vi "3ph Power from 9239 (DAQmx).vi"(5 "PTO1 Summary":refnum<queue>, 7 "PTO1 TDMS":refnum<queue>, 8 "error in":errorcluster, 10 "3ph Inputs":T1={"voltage channels"="Mod3/ai0:2", "minimum voltage value"=-10.0, "maximum voltage value"=10.0, "3ph sample rate [Hz]"=5000.0, "3phf samples per channel"=500, "Voltage Scaling"=100.0, "Current Scaling"=100.0} {"Current Scaling" format="%0.2f"; "Voltage Scaling" format="%0.2f"; "3phf samples per channel" format="%0.2f"; "3ph sample rate [Hz]" format="%0.2f"; "maximum voltage value" format="%0.2f"; "minimum voltage value" format="%0.2f"}, 11 "Queue in":refnum<queue>) -> (0 "error out":errorcluster)   [LabVIEW 2019]
doc: "Demonstrates how to implement basic power measurement on a three-phase electrical power system, such as power and energy values, frequency amplitudes, and symmetrical components."
uses:
  3ph Inputs.ctl
  Globals and Definitions/System Message.ctl
  <vilib>/DAQmx/read.llb/DAQmx Read (Analog 1D Wfm NChan NSamp).vi
  <vilib>/DAQmx/create/channels.llb/DAQmx Create Channel (AI-Voltage-Basic).vi
  <vilib>/DAQmx/configure/timing.llb/DAQmx Timing (Sample Clock).vi
  Globals and Definitions/Initialization Globals.vi
  Globals and Definitions/RT Globals RD v1.0.vi
  <vilib>/DAQmx/miscellaneous.llb/DAQmx Fill In Error Info.vi
  Globals and Definitions/Control Globals RD v1.0.vi
  <vilib>/addons/Electrical Power/Basic/Measurement/Frequency (N Channels).vi
  <vilib>/addons/Electrical Power/Basic/Measurement/RMS (N Channels).vi
  <vilib>/addons/Electrical Power/Basic/Measurement/Power (N Channels).vi
  <vilib>/addons/Electrical Power/Basic/Measurement/Energy (N Channels).vi
  <vilib>/addons/Electrical Power/Basic/NI_EP_Basic.lvlib
  <resource>/objmgr/daqmx.rc
panel:
  out "Current":waveform(dbl)[](graph)
  out "Voltages":waveform(dbl)[](graph)
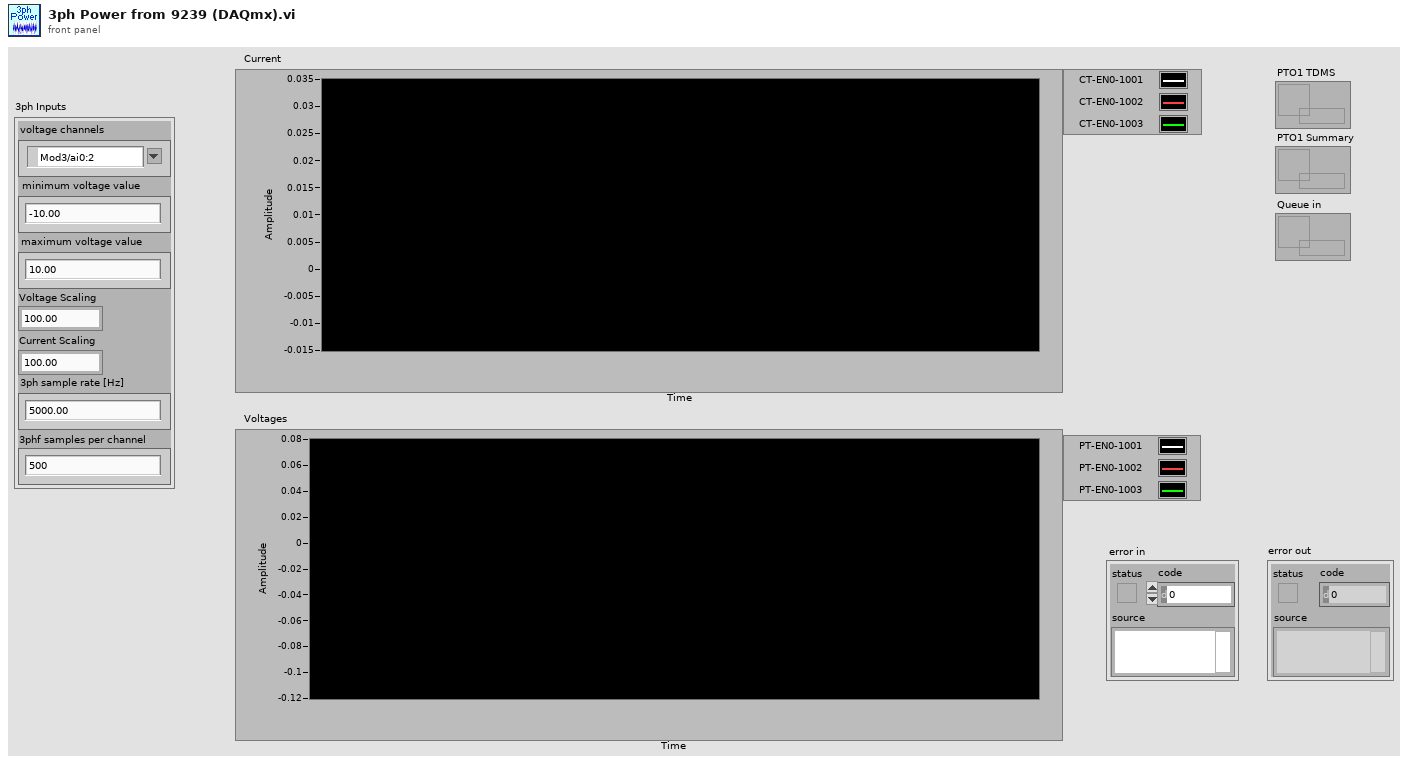
[diagram p1: front panel]
types:
  T1 = typedef "3ph Inputs.ctl" = cluster{"voltage channels":tag, "minimum voltage value":dbl, "maximum voltage value":dbl, "3ph sample rate [Hz]":dbl, "3phf samples per channel":i32, "Voltage Scaling":dbl, "Current Scaling":dbl}
  T2 = typedef "NI_EP_Basic.lvlib/basic_Power Value.ctl" = cluster{"active power [W]":dbl, "apparent power [VA]":dbl, "reactive power [VAR]":dbl, "power factor":dbl}
  T3 = typedef "NI_EP_Basic.lvlib/basic_Energy Value.ctl" = cluster{"active energy [Wh]":dbl, "apparent energy [VAh]":dbl, "reactive energy [VARh]":dbl}
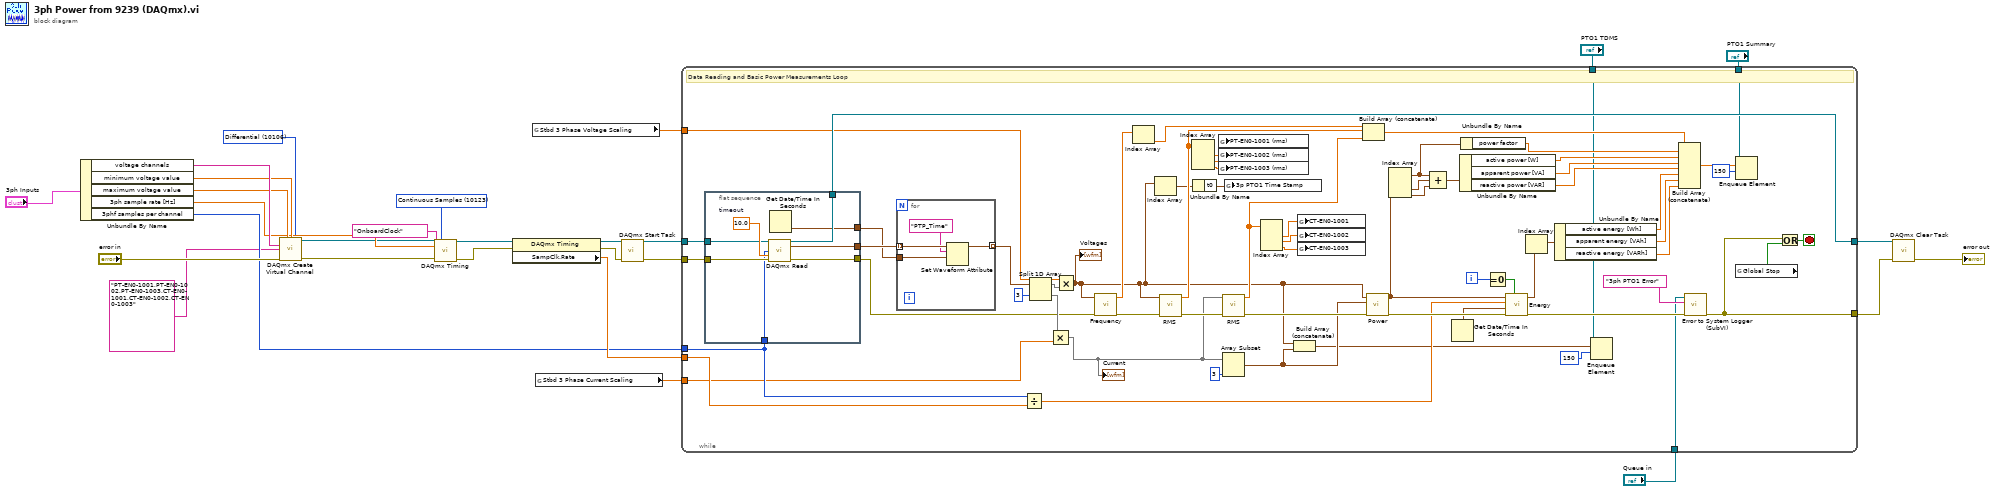
[diagram p0: block diagram]
diagram:
  w10 = 10106 items=["Default"=-1, "RSE"=10083, "NRSE"=10078, "Differential"=10106, "Pseudodifferential"=12529] ("input terminal configuration")
  w26 = 10123 items=["Finite Samples"=10178, "Continuous Samples"=10123] ("sample mode")
  n1 = Unbundle By Name("3ph Inputs") -> ("voltage channels"=w17:tag, "minimum voltage value"=w16:dbl, "maximum voltage value"=w15:dbl, "3ph sample rate [Hz]"=w14:dbl, "3phf samples per channel"=w13:i32)
  n2 = call-poly <vilib>:"DAQmx Create Virtual Channel.vi"("maximum value"=w15, "minimum value"=w16, "input terminal configuration"=w10, "physical channels"=w17, "name to assign"="PT-EN0-1001,PT-EN0-1002,PT-EN0-1003,CT-EN0-1001,CT-EN0-1002,CT-EN0-1003", "error in"="error in") -> ("task out"=w12:refnum<k21>, "error out"=w11:errorcluster)  [unwired: 8 in]
  n3 = call-poly <vilib>:"DAQmx Timing.vi"("task/channels in"=w12, "sample mode"=w26, "rate"=w14, "source"=tag "OnboardClock", "error in"=w11) -> ("task out"=w24:refnum<k21>, "error out"=w22:errorcluster)  [unwired: 9 in]
  n4 = property class="DAQmx Timing"(reference=w24, error in=w22) -> (reference out=w23:refnum<k21>, error out=w21:errorcluster, "SampClk.Rate"=w20:dbl)
  n5 = global read "Initialization Globals.vi" "Stbd 3 Phase Voltage Scaling"() -> (w8:dbl[])
  n6 = global read "Initialization Globals.vi" "Stbd 3 Phase Current Scaling"() -> (w7:dbl[])
  n7 = call <vilib>:"DAQmx Start Task.vi"("task/channels in"=w23, "error in"=w21) -> ("task out"=w28:refnum<k21>, "error out"=w25:errorcluster)  [unwired: 12 in]
  n8 = while {
    tunnel: w28 -> [w38]
    tunnel: [w91] -> w27
    tunnel: w20 -> [w60]
    tunnel: w13 -> [w59]
    tunnel: w8 -> [w32]
    tunnel: w7 -> [w48]
    tunnel: "PTO1 Summary" -> [w46]
    tunnel: "PTO1 TDMS" -> [w39]
    tunnel: w25 -> [w92]
    tunnel: "Queue in" -> [w40]
    tunnel: [w29] -> w1
    i -> [w58]
    stop <- w93 stop-if-true
    # "Data Reading and Basic Power Measurements Loop"
    n9 = flat-sequence {
      tunnel: w92 -> [w101]
      tunnel: [w100] -> w91
      tunnel: [w95] -> w35
      tunnel: [w98] -> w61
      tunnel: w59 -> [w97]
      tunnel: w38 -> [w96]
      tunnel: [w94] -> w31
      frame #0 {
        w99 = 10.0  # timeout
        n10 = call-poly <vilib>:"DAQmx Read.vi"("task/channels in"=w96, "number of samples per channel"=w97, "timeout"=w99, "error in"=w101) -> ("task out"=w100:refnum<k21>, "data"=w95:waveform(dbl)[], "error out"=w98:errorcluster)  [unwired: 9 in]
        n11 = Get Date/Time In Seconds() -> (seconds since 1Jan1904=w94:timestamp)
      }
    }
    n12 = for {
      tunnel: w35 -> [w105] mode=indexing
      tunnel: w31 -> [w104]
      tunnel: [w103] -> w30 mode=indexing
      n13 = Set Waveform Attribute(5:w104, 6:"PTP_Time" ("name"), 7:w105) -> (3:w103:waveform(dbl))  [unwired: 1 in, 2 out]
    }
    n14 = Divide(x=w59, y=w60) -> (x/y=w85:dbl)
    n15 = Split 1D Array(array=w30, index=3) -> (first subarray=w80:waveform(dbl)[], second subarray=w79:waveform(dbl)[])
    n16 = Multiply(x=w79, y=w48) -> (x*y=w33:waveform(dbl)[])
    "Current" <- w33
    n17 = Multiply(x=w32, y=w80) -> (x*y=w34:waveform(dbl)[])
    "Voltages" <- w34
    n18 = call-poly <vilib>:"Frequency.vi"("error in (no error)"=w61, "waveforms"=w34) -> ("error out"=w90:errorcluster, "frequencies"=w89:dbl[])  [unwired: 8 in]
    n19 = Index Array(array=w89) -> (element=w74:dbl)  [unwired: 1 in]
    n20 = Index Array(array=w34) -> (element=w53:waveform(dbl))  [unwired: 1 in]
    n21 = call-poly <vilib>:"RMS.vi"("error in (no error)"=w90, "waveforms"=w34) -> ("error out"=w83:errorcluster, "RMS values"=w54:dbl[])  [unwired: 8 in]
    n22 = Index Array(array=w54) -> (element #1=w57:dbl, element #2=w56:dbl, element #3=w55:dbl)  [unwired: 3 in]
    n23 = Unbundle By Name(w53) -> ("t0"=w47:timestamp)
    n24 = global write "Control Globals RD v1.0.vi" "PT-EN0-1001 (rms)"(w57) -> ()
    n25 = global write "Control Globals RD v1.0.vi" "PT-EN0-1002 (rms)"(w56) -> ()
    n26 = global write "Control Globals RD v1.0.vi" "PT-EN0-1003 (rms)"(w55) -> ()
    n27 = Array Subset(array=w33, length=3) -> (w78:waveform(dbl)[])  [unwired: 1 in]
    n28 = call-poly <vilib>:"RMS.vi"("error in (no error)"=w83, "waveforms"=w33) -> ("error out"=w82:errorcluster, "RMS values"=w49:dbl[])  [unwired: 8 in]
    n29 = global write "Control Globals RD v1.0.vi" "3p PTO1 Time Stamp"(w47) -> ()
    n30 = Index Array(array=w49) -> (element #1=w52:dbl, element #2=w51:dbl, element #3=w50:dbl)  [unwired: 3 in]
    n31 = Build Array (concatenate)(w34, w78) -> (w43:waveform(dbl)[])
    n32 = global write "Control Globals RD v1.0.vi" "CT-EN0-1001"(w52) -> ()
    n33 = global write "Control Globals RD v1.0.vi" "CT-EN0-1002"(w51) -> ()
    n34 = global write "Control Globals RD v1.0.vi" "CT-EN0-1003"(w50) -> ()
    n35 = Build Array (concatenate)(w74, w54, w49) -> (w73:dbl[])
    n36 = call-poly <vilib>:"Power.vi"("error in (no error)"=w82, "current waveforms"=w78, "voltage waveforms"=w34) -> ("error out"=w88:errorcluster, "power values"=w77:T2[])  [unwired: 7 in]
    n37 = Index Array(array=w77) -> (element #1=w66:T2, element #2=w69:T2, element #3=w68:T2)  [unwired: 3 in]
    n38 = Compound Arithmetic op=ADD(w66, w69, w68) -> (w67:T2)
    n39 = Get Date/Time In Seconds() -> (seconds since 1Jan1904=w87:timestamp)
    n40 = Unbundle By Name(w67) -> ("active power [W]"=w62:dbl, "apparent power [VA]"=w64:dbl, "reactive power [VAR]"=w63:dbl)
    n41 = Unbundle By Name(w66) -> ("power factor"=w65:dbl)
    n42 = Equal To 0?(x=w58) -> (x = 0?=w86:bool)
    n43 = call-poly <vilib>:"Energy.vi"("reset? (F)"=w86, "error in (no error)"=w88, "start timestamp"=w87, "interval length [s]"=w85, "power values"=w77) -> ("error out"=w42:errorcluster, "energy values"=w76:T3[])  [unwired: 4 in, 1 out]
    n44 = Index Array(array=w76) -> (element=w75:T3)  [unwired: 1 in]
    n45 = Unbundle By Name(w75) -> ("active energy [Wh]"=w72:dbl, "apparent energy [VAh]"=w71:dbl, "reactive energy [VARh]"=w70:dbl)
    n46 = Enqueue Element(queue=w39, element=w43, timeout in ms (-1)=150) -> ()  [unwired: 1 in, 3 out]
    n47 = Build Array (concatenate)(w73, w65, w62, w64, w63, w72, w71, w70) -> (w44:dbl[])
    n48 = call "Error to System Logger (SubVI).vi"("error in (no error)"=w42, "Message Tag"="3ph PTO1 Error", "Sys Msg Queue"=w40) -> ("error out"=w29:errorcluster)  [unwired: 8 in]
    n49 = Enqueue Element(queue=w46, element=w44, timeout in ms (-1)=150) -> ()  [unwired: 1 in, 3 out]
    n50 = global read "RT Globals RD v1.0.vi" "Global Stop"() -> (w45:bool)
    n51 = Or(x=w29, y=w45) -> (x .or. y?=w93:bool)
  }
  n52 = call <vilib>:"DAQmx Clear Task.vi"("task in"=w27, "error in"=w1) -> ("error out"=→"error out":errorcluster)  [unwired: 13 in]
